vi "getCost.vi"(8 "error in (no error)":errorcluster, 11 "CondimentDecorator in":refnum<class "CondimentDecorator.lvclass">) -> (0 "error out":errorcluster, 2 "cost":dbl, 3 "CondimentDecorator out":refnum<class "CondimentDecorator.lvclass">)   [LabVIEW 2017, in "CondimentDecorator.lvclass"]
uses:
  CondimentDecorator.lvclass
  Beverage Class/Beverage.lvclass
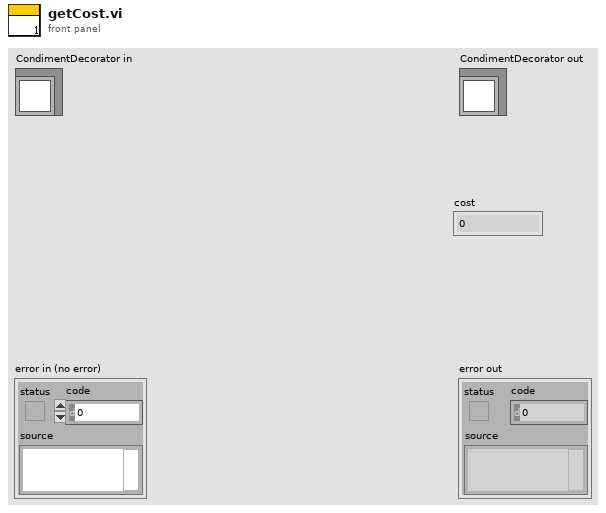
[diagram p1: front panel]
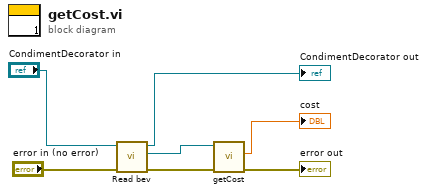
[diagram p0: block diagram]
diagram:
  n1 = call-dynamic "Read bev.vi"("error in (no error)"="error in (no error)", "CondimentDecorator in"="CondimentDecorator in") -> ("error out"=w6:errorcluster, "Beverage.lvclass"=w2:refnum<class "Beverage.lvclass">, "CondimentDecorator out"=→"CondimentDecorator out":refnum<class "CondimentDecorator.lvclass">)  [unwired: 7 in]
  n2 = call-dynamic "getCost.vi"("error in (no error)"=w6, "Beverage in"=w2) -> ("error out"=→"error out":errorcluster, "cost"=→"cost":dbl)  [unwired: 7 in, 1 out]
